vi "Array 16bit To 24bit.vi"(11 "Unsigned Byte Array":u8[](array[numeric])) -> (3 "Appended Array":u8[](array[numeric]))   [LabVIEW 2009, in "DSO1K.lvlib"]
doc: "The 16 bit data into the 24 bit data."
uses:
  <instrlib>/DSO1K/DSO1K.lvlib
panel:
  in  "8bit Cluster":T1
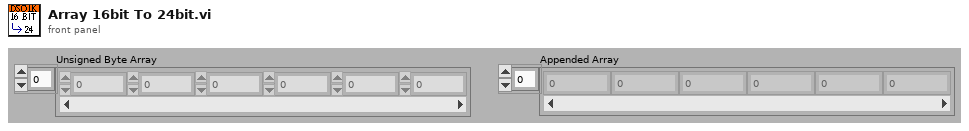
[diagram p1: front panel]
types:
  T1 = cluster{"bit 1":bool, "bit 2":bool, "bit 3":bool, "bit 4":bool, "bit 5":bool, "bit 6":bool, "bit 7":bool, "bit 8":bool}
  T2 = cluster{"Boolean array[0]":bool, "Boolean array[1]":bool, "Boolean array[2]":bool, "Boolean array[3]":bool, "Boolean array[4]":bool, "Boolean array[5]":bool, "Boolean array[6]":bool, "Boolean array[7]":bool, "Boolean array[8]":bool, "Boolean array[9]":bool, "Boolean array[10]":bool, "Boolean array[11]":bool, "Boolean array[12]":bool, "Boolean array[13]":bool, "Boolean array[14]":bool, "Boolean array[15]":bool}
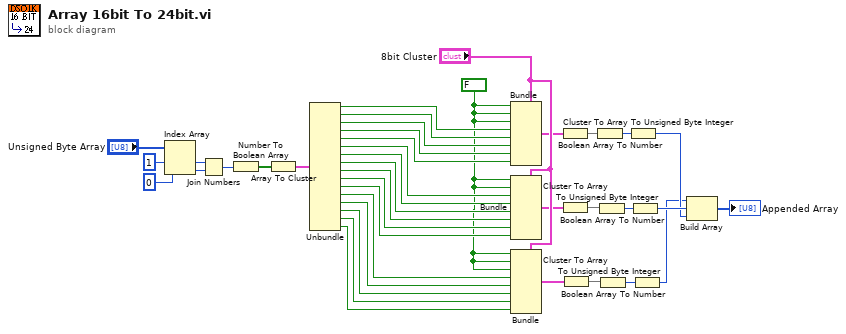
[diagram p0: block diagram]
diagram:
  w3 = FALSE
  n1 = Index Array(array="Unsigned Byte Array", index #1=1 ("index"), index #2=0 ("index")) -> (element #1=w27:u8, element #2=w26:u8)
  n2 = Join Numbers(hi=w27, lo=w26) -> ((hi.lo)=w35:u16)
  n3 = Number To Boolean Array(number=w35) -> (Boolean array=w37:bool[])
  n4 = Array To Cluster(array=w37) -> (cluster=w36:T2)
  n5 = Unbundle(w36) -> ("Boolean array[0]"=w4:bool, "Boolean array[1]"=w5:bool, "Boolean array[2]"=w6:bool, "Boolean array[3]"=w7:bool, "Boolean array[4]"=w8:bool, "Boolean array[5]"=w9:bool, "Boolean array[6]"=w10:bool, "Boolean array[7]"=w11:bool, "Boolean array[8]"=w12:bool, "Boolean array[9]"=w13:bool, "Boolean array[10]"=w14:bool, "Boolean array[11]"=w15:bool, "Boolean array[12]"=w16:bool, "Boolean array[13]"=w17:bool, "Boolean array[14]"=w18:bool, "Boolean array[15]"=w19:bool)
  n6 = Bundle(cluster="8bit Cluster", "bit 1"=w3, "bit 2"=w3, "bit 3"=w3, "bit 4"=w4, "bit 5"=w5, "bit 6"=w6, "bit 7"=w7, "bit 8"=w8) -> (w33:T1)
  n7 = Bundle(cluster="8bit Cluster", "bit 1"=w3, "bit 2"=w3, "bit 3"=w9, "bit 4"=w10, "bit 5"=w11, "bit 6"=w12, "bit 7"=w13, "bit 8"=w14) -> (w31:T1)
  n8 = Bundle(cluster="8bit Cluster", "bit 1"=w3, "bit 2"=w3, "bit 3"=w3, "bit 4"=w15, "bit 5"=w16, "bit 6"=w17, "bit 7"=w18, "bit 8"=w19) -> (w28:T1)
  n9 = Cluster To Array(cluster=w33) -> (array=w32:bool[])
  n10 = Cluster To Array(cluster=w31) -> (array=w30:bool[])
  n11 = Cluster To Array(cluster=w28) -> (array=w29:bool[])
  n12 = Boolean Array To Number(Boolean array=w32) -> (number=w23:u32)
  n13 = Boolean Array To Number(Boolean array=w30) -> (number=w24:u32)
  n14 = Boolean Array To Number(Boolean array=w29) -> (number=w25:u32)
  n15 = To Unsigned Byte Integer(number=w23) -> (unsigned 8bit integer=w2:u8)
  n16 = To Unsigned Byte Integer(number=w24) -> (unsigned 8bit integer=w22:u8)
  n17 = To Unsigned Byte Integer(number=w25) -> (unsigned 8bit integer=w1:u8)
  n18 = Build Array(w1, w22, w2) -> (→"Appended Array":u8[])
